vi "Update.vi"(8 "error in (no error)":errorcluster, 10 "Square Colors":u32[][](array[colorbox]), 11 "Square Field Panel in":refnum<class "Square Field Panel.lvclass">) -> (0 "error out":errorcluster, 3 "Square Field Panel out":refnum<class "Square Field Panel.lvclass">)   [LabVIEW 2020, in "SB App.lvlib" / "Square Field Panel.lvclass"]
uses:
  Square Field Panel.lvclass
  Square Field Panel.lvclass/Square Field Panel.ctl
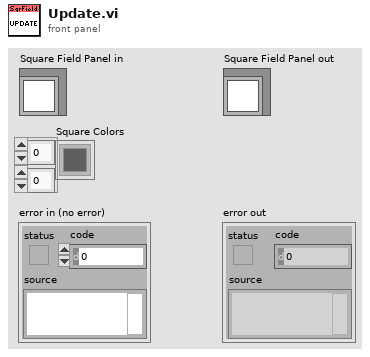
[diagram p1: front panel]
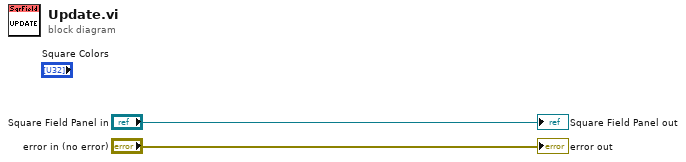
[diagram p0: block diagram]
diagram:
  "error out" <- "error in (no error)"
  "Square Field Panel out" <- "Square Field Panel in"
